vi "TDTRX6-Wait For Buffer Space.vi"(0 "RPcox":refnum<k7>, 5 "Next Buffer":i32, 7 "Tag":string="ch2Index", 9 "Buffer Length":i32, 11 "error in (no error)":errorcluster) -> (4 "RPcox Out":refnum<k7>, 6 "Next Buffer Out":i32, 15 "error out":errorcluster)   [LabVIEW 2020]
uses:
  TDT-Globals.vi
panel:
  out "Available":bool
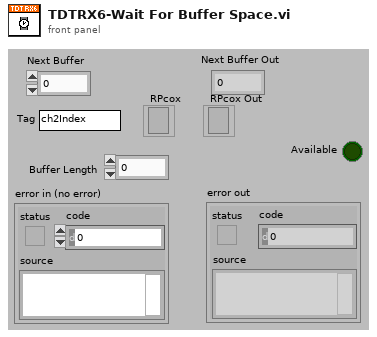
[diagram p1: front panel]
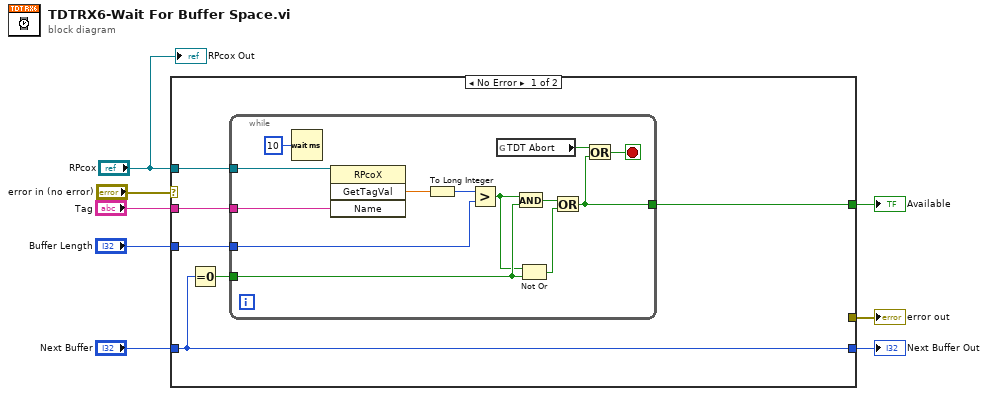
[diagram p0: block diagram]
diagram:
  n1 = case shown="No Error" "error in (no error)" {
    selector: "error in (no error)" -> [_ w28]
    tunnel: [_ w28] -> w7
    tunnel: "RPcox" -> [w14 _]
    tunnel: "Buffer Length" -> [w13 _]
    tunnel: "Next Buffer" -> [w10 _]
    tunnel: [w11 _] -> w4
    tunnel: [w10 _] -> w3
    tunnel: "Tag" -> [w9 _]
    frame No Error {
      n2 = Equal To 0?(x=w10) -> (x = 0?=w12:bool)
      n3 = while {
        tunnel: w14 -> [w27]
        tunnel: w13 -> [w24]
        tunnel: w12 -> [w22]
        tunnel: [w18] -> w11
        tunnel: w9 -> [w15]
        stop <- w17 stop-if-true
        n4 = Wait (ms)(milliseconds to wait=u32 10) -> ()  [unwired: 1 out]
        n5 = invoke class="RPcoX" method="GetTagVal"(reference=w27, "Name"=w15) -> ("GetTagVal"=w26:sgl)  [unwired: 2 in, 3 out]
        n6 = To Long Integer(number=w26) -> (32bit integer=w25:i32)
        n7 = Greater?(x=w25, y=w24) -> (0:w21:bool)
        n8 = global read "TDT-Globals.vi" "TDT Abort"() -> (w19:bool)
        n9 = And(x=w21, y=w22) -> (x .and. y?=w23:bool)
        n10 = Not Or(1:w22, 2:w21) -> (0:w20:bool)
        n11 = Or(x=w23, y=w20) -> (x .or. y?=w18:bool)
        n12 = Or(x=w19, y=w18) -> (x .or. y?=w17:bool)
      }
    }
    frame Error {
    }
  }
  "error out" <- w7
  "Next Buffer Out" <- w3
  "Available" <- w4
  "RPcox Out" <- "RPcox"
